vi "showHolo.vi"(7 "Window Number (0...15)":u16=1, 8 "error in (no error)":errorcluster, 9 "active?":bool=TRUE, 11 "Image":T1=refnum) -> (0 "error out":errorcluster, 1 "Windows title":string, 3 "Image Out (duplicate)":T1)   [LabVIEW 2023]
uses:
  <vilib>/vision/Image Controls.llb/IMAQ Image.ctl
panel:
  in  "Scrollbars":i32(ring)=2 items=["Hide", "Show", "No change"]
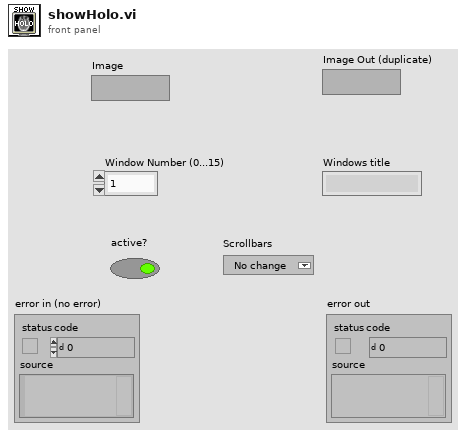
[diagram p1: front panel]
types:
  T1 = typedef "IMAQ Image.ctl" = refnum<image>
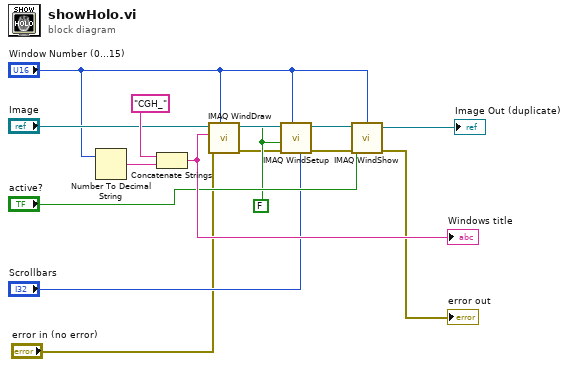
[diagram p0: block diagram]
diagram:
  w5 = FALSE ("Window can grow? (Yes)")
  n1 = Number To Decimal String(number="Window Number (0...15)") -> (decimal integer string=w12:string)  [unwired: 1 in]
  n2 = Concatenate Strings("CGH_" ("Title"), w12) -> (w11:string)
  "Windows title" <- w11
  n3 = call "IMAQ WindDraw"("Window Number (0...15)"="Window Number (0...15)", "error in (no error)"="error in (no error)", "Title"=w11, "Image"="Image") -> ("error out"=w4:errorcluster, "Image Out (duplicate)"=→"Image Out (duplicate)":T1)  [unwired: 6 in]
  n4 = call "IMAQ WindSetup"("Scrollbars (No change)"="Scrollbars", "Window Number (0...15)"="Window Number (0...15)", "error in (no error)"=w4, "Window has title bar? (Yes)"=w5, "Window can grow? (Yes)"=w5) -> ("error out"=w3:errorcluster)  [unwired: 6 in]
  n5 = call "IMAQ WindShow"("error in (no error)"=w3, "Hide/Show (Show)"="active?", "Window Number (0...15)"="Window Number (0...15)") -> ("error out"=→"error out":errorcluster)  [unwired: 3 in, 2 out]
